vi "Get Curr and Volt.vi"(0 "PS_Sim in":refnum<class "PS Simulated.lvclass">, 11 "error in (no error)":errorcluster) -> (4 "PS_Sim out":refnum<class "PS Simulated.lvclass">, 6 "Voltage":dbl, 8 "Current":dbl, 10 "Output?":bool, 15 "error out":errorcluster)   [LabVIEW 2021, in "PS.lvlib" / "PS Simulated.lvclass"]
uses:
  PS Simulated.lvclass
  PS Simulated.lvclass/PS Simulated.ctl
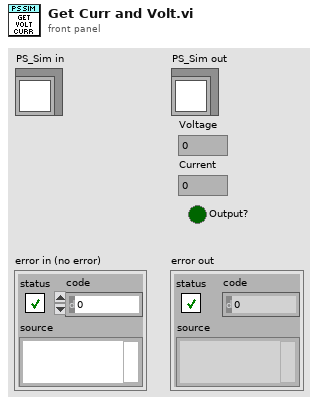
[diagram p1: front panel]
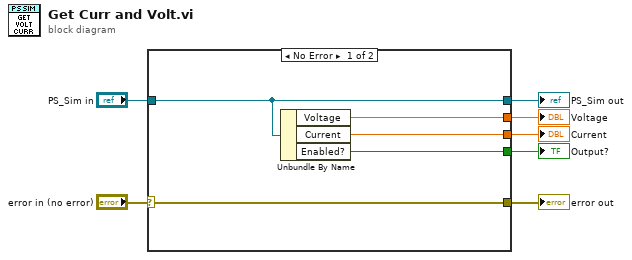
[diagram p0: block diagram]
diagram:
  n1 = case shown="No Error" "error in (no error)" {
    selector: "error in (no error)" -> [w12 w13]
    tunnel: [w11 w14] -> w6
    tunnel: "PS_Sim in" -> [w11 w14]
    tunnel: [w12 w13] -> w4
    tunnel: [w10 _] -> w3
    tunnel: [w9 _] -> w2
    tunnel: [w8 _] -> w1
    frame No Error {
      n2 = Unbundle By Name(w11) -> ("Voltage"=w10:dbl, "Current"=w9:dbl, "Enabled?"=w8:bool)
    }
    frame Error {
    }
  }
  "error out" <- w4
  "PS_Sim out" <- w6
  "Current" <- w2
  "Voltage" <- w3
  "Output?" <- w1
